vi "sns subscription sample.vi"() -> ()   [LabVIEW 2015]
uses:
  Subscription/Subscription Protocol.ctl
  Core/HTTP Request/AWS Credentials.ctl
  Core/HTTP Request/Region.ctl
  Topic/Mutable Topic Attribute Value Pair.ctl
  Topic/Mutable Topic Attribute.ctl
  Subscription/Subscription.lvclass/Subscription.ctl
  Core/ARN/ARN.lvclass/ARN.ctl
  Core/ARN/Read ARN.vi
  Subscription/Read Endpoint.vi
  Subscription/Read Owner.vi
  Subscription/Read Protocol.vi
  Subscription/Read Topic.vi
  Topic/Topic.lvclass
  Subscription/Subscription.lvclass
  Core/HTTP Request/HTTP Request.lvclass
panel:
  out "Owner":string
  out "Protocol":T1
  out "subscription ARLs":string[](array[string])
  out "subscription names":string[](array[string])
  out "topic ARN":string
  out "Endpoint":string
  out "found?":bool
  out "topic names":string[](array[string])
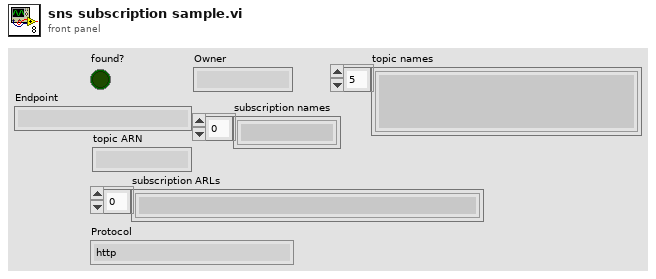
[diagram p1: front panel]
types:
  T1 = typedef "NI_AWS_SNS.lvlib/Subscription.lvclass/Subscription Protocol.ctl" = enum16{"http", "https", "email", "email-json", "sms", "sqs", "application", "lambda"}
  T2 = typedef "NI_AWS_SNS.lvlib/Topic.lvclass/Mutable Topic Attribute Value Pair.ctl" = cluster{"Attribute":T3, "Value":string}
  T3 = typedef "NI_AWS_SNS.lvlib/Topic.lvclass/Mutable Topic Attribute.ctl" = enum16{"Policy", "DisplayName", "DeliveryPolicy"}
  T4 = typedef "NI_AWS_Core.lvlib/HTTP Request.lvclass/Region.ctl" = enum16{"us-east-1", "us-east-2", "us-west-1", "us-west-2", "ap-northeast-1", "ap-northeast-2", "ap-southeast-1", "ap-southeast-2", "ca-central-1", "eu-central-1", "eu-west-1", "eu-west-2", "sa-east-1"}
  T5 = typedef "NI_AWS_Core.lvlib/HTTP Request.lvclass/AWS Credentials.ctl" = cluster{"Access Key":string, "Secret Key":string}
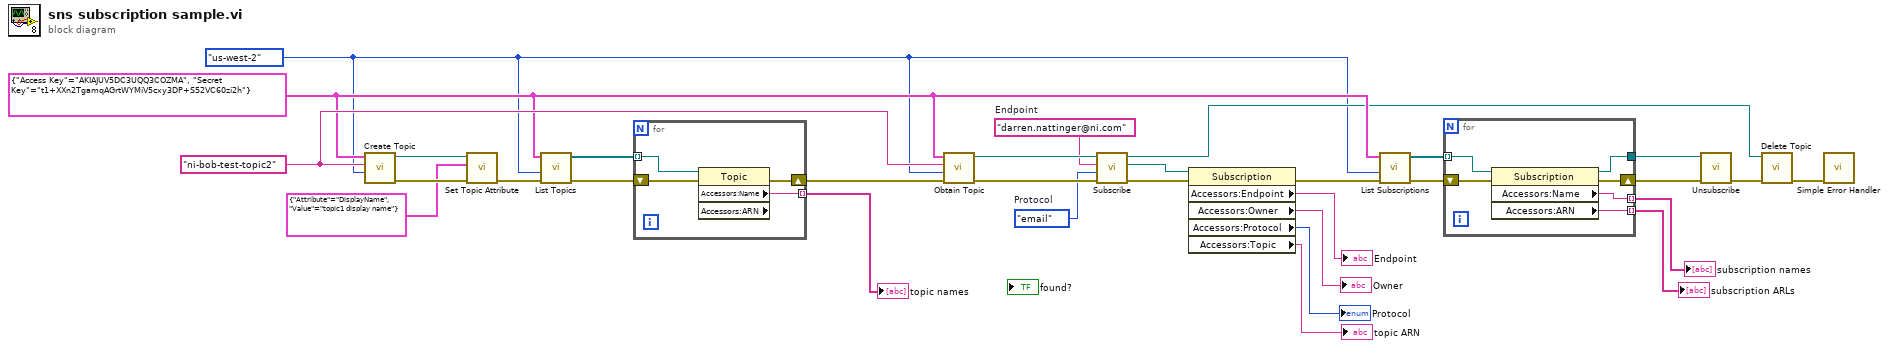
[diagram p0: block diagram]
diagram:
  w9 = Subscription_Protocol."email"  # Protocol
  w23 = "ni-bob-test-topic2" ("Name")
  w1 = Region."us-west-2" ("Region")
  w20 = T5 {"Access Key"="AKIAJUV5DC3UQQ3COZMA", "Secret Key"="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"} ("AWS Credentials")
  w10 = "darren.nattinger@ni.com"  # Endpoint
  n1 = call "Create Topic.vi"("Region"=w1, "Name"=w23, "AWS Credentials"=w20) -> ("error out"=w30:errorcluster, "Topic out"=w31:refnum<class "Topic.lvclass">)  [unwired: 7 in]
  n2 = call "Set Topic Attribute.vi"("error in (no error)"=w30, "Topic Attribute"=T2 {"Attribute"=enum."DisplayName", "Value"="topic1 display name"}, "Topic"=w31) -> ("error out"=w28:errorcluster)  [unwired: 7 in, 1 out]
  n3 = call "List Topics.vi"("error in (no error)"=w28, "Region"=w1, "AWS Credentials"=w20) -> ("error out"=w26:errorcluster, "Topics out"=w27:refnum<class "Topic.lvclass">[])  [unwired: 7 in]
  n4 = for {
    tunnel: w27 -> [w35] mode=indexing
    shift-right: [w33] -> w24
    shift-left: w26 -> [w34]
    tunnel: [w32] -> w25 mode=indexing
    n5 = property class="Topic" props=["Accessors:Name", "Accessors:ARN"](reference=w35, error in=w34) -> (error out=w33:errorcluster, "Accessors:Name"=w32:string)  [unwired: 2 out]
  }
  "topic names" <- w25
  n6 = call "Obtain Topic.vi"("error in (no error)"=w24, "Region"=w1, "Name"=w23, "AWS Credentials"=w20) -> ("error out"=w22:errorcluster, "Topic out"=w13:refnum<class "Topic.lvclass">)  [unwired: 6 in]
  n7 = call "Subscribe.vi"("error in (no error)"=w22, "Protocol"=w9, "Endpoint"=w10, "Topic in"=w13) -> ("error out"=w8:errorcluster, "Subscription"=w11:refnum<class "Subscription.lvclass">, "Topic out"=w12:refnum<class "Topic.lvclass">)  [unwired: 5 in]
  n8 = property class="Subscription"(reference=w11, error in=w8) -> (error out=w21:errorcluster, "Accessors:Endpoint"=→"Endpoint":string, "Accessors:Owner"=→"Owner":string, "Accessors:Protocol"=→"Protocol":T1, "Accessors:Topic"=→"topic ARN":string)  [unwired: 1 out]
  n9 = call "List Subscriptions.vi"("error in (no error)"=w21, "Region"=w1, "AWS Credentials"=w20) -> ("error out"=w16:errorcluster, "Subscriptions out"=w17:refnum<class "Subscription.lvclass">[])  [unwired: 7 in]
  n10 = for {
    tunnel: w17 -> [w41] mode=indexing
    shift-right: [w39] -> w15
    shift-left: w16 -> [w40]
    tunnel: [w38] -> w14 mode=indexing
    tunnel: [w37] -> w7 mode=indexing
    tunnel: [w36] -> w2
    n11 = property class="Subscription"(reference=w41, error in=w40) -> (reference out=w36:refnum<class "Subscription.lvclass">, error out=w39:errorcluster, "Accessors:Name"=w38:string, "Accessors:ARN"=w37:string)
  }
  "subscription names" <- w14
  "subscription ARLs" <- w7
  n12 = call "Unsubscribe.vi"("error in (no error)"=w15, "Subscription"=w2) -> ("error out"=w19:errorcluster)  [unwired: 9 in]
  n13 = call "Delete Topic.vi"("error in (no error)"=w19, "Topic"=w12) -> ("error out"=w18:errorcluster)  [unwired: 9 in]
  n14 = call <vilib>:"Simple Error Handler.vi"("error in (no error)"=w18) -> ()  [unwired: 4 in, 5 out]
